vi "诊断标定3.vi"(8 "CAN端口":u16(ring), 9 "设备索引号":u16(ring), 10 "CAN卡类型":u32(ring)=21) -> ()   [LabVIEW 2013] (continued)
                        n4317 = Build Array(string[] ["电池生产日期", "电池厂商", "电池类型", "电池包组号", "电池包产权标识", "电池包应用车型", "电池串联", "电池并联", "累计充电总安时", "累计放电总安时", "电池包额定容量", "电池包额定能量", "电池包额定总电压", "电池充满次数", "电池放空次数", "电池充电次数", "实际容量"], w6126) -> (w6147:string[][])
                        n4318 = Transpose 2D Array(2D array=w6147) -> (transposed array=w6125:string[][])
                      }
                    }
                    n4319 = Insert Into Array(array=w5966, index (col)=2 ("禁用的索引 (列)"), new element #1=w5963, new element #2=w5962, new element #3=w5961, new element #4=w5960, new element #5=w5959) -> (w5964:string[][])  [unwired: 1 in]
                  }
                  frame "从板" {
                    n4320 = local read "从板号"() -> (w6163:u8)
                    n4321 = Number To Decimal String(number=w6163) -> (decimal integer string=w6160:string)  [unwired: 1 out]
                    n4322 = Concatenate Strings("S", w6160) -> (w6161:string)
                    n4323 = Build Array("从板号" ("元素"), w6160) -> (w6158:string[])
                    n4324 = stacked-sequence {
                      seq-local: [string[] ["风机开启温度", "风机关闭温度", "加热开启温度", "加热关闭温度", "风机开启温差", "风机关闭温差", "加热关闭温差"] _ _ _ _ _] -> [_ _ _ w6232 _ _]
                      seq-local: [w6175 _ _ _ _ _] -> [_ _ _ w6228 _ _]
                      seq-local: [_ string[] ["电压过高一级", "电压过低一级", "温度过高一级", "温度过低一级", "电压不均衡一级", "温度不均衡一级", "SOC过低一级"] _ _ _ _] -> [_ _ _ w6231 _ _]
                      seq-local: [_ w6193 _ _ _ _] -> [_ _ _ w6227 _ _]
                      seq-local: [_ _ string[] ["电压过高二级", "电压过低二级", "温度过高二级", "温度过低二级", "电压不均衡二级", "温度不均衡二级", "SOC过低二级"] _ _ _] -> [_ _ _ w6230 _ _]
                      seq-local: [_ _ w6208 _ _ _] -> [_ _ _ w6226 _ _]
                      tunnel: w6158 -> [w6188 _ _ _ _ _]
                      tunnel: [w6177 _ _ _ _ _] -> w6156
                      tunnel: [_ _ _ w6233 _ _] -> w6154
                      tunnel: [_ _ _ _ w6271 _] -> w6153
                      tunnel: [_ _ _ _ _ w6307] -> _
                      frame #0 {
                        w6168 = string[] ["", "", "", "", "", "", "", "", "", "", "  "]
                        n4325 = control-ref of="项目信息 2"() -> (w6187:refnum<vi>)
                        n4326 = property class="Tbl (严格)"(reference=w6187) -> ("Value"=w6165:string[][])  [unwired: 1 in, 2 out]
                        n4327 = control-ref of="加热控制参数"() -> (w6179:refnum<vi>)
                        n4328 = property class="Clust (严格)"(reference=w6179) -> ("Value"=w6186:T11)  [unwired: 1 in, 2 out]
                        n4329 = Unbundle(w6186) -> ("风机开启温度"=w6185:dbl, "风机关闭温度"=w6184:dbl, "加热开启温度"=w6183:dbl, "加热关闭温度"=w6182:dbl, "风机开启温差"=w6181:dbl, "风机关闭温差"=w6180:dbl, "加热关闭温差"=w6174:dbl)
                        n4330 = Build Array(w6185, w6184, w6183, w6182, w6181, w6180, w6174) -> (w6178:dbl[])
                        n4331 = for {
                          tunnel: w6178 -> [w6191] mode=indexing
                          tunnel: [w6190] -> w6175 mode=indexing
                          n4332 = Format Into String(format string="%#f" ("格式字符串"), w6191) -> (resulting string=w6190:string)  [unwired: 2 in, 1 out]
                        }
                        n4333 = Index Array(array=w6165, index (col)=0 ("禁用的索引 (列)")) -> (element=w6172:string[])  [unwired: 1 in]
                        n4334 = Index Array(array=w6165, index (col)=1 ("禁用的索引 (列)")) -> (element=w6171:string[])  [unwired: 1 in]
                        n4335 = Insert Into Array(array=w6172, new element=w6168) -> (w6170:string[])  [unwired: 1 in]
                        n4336 = Insert Into Array(array=w6171, new element=w6168) -> (w6169:string[])  [unwired: 1 in]
                        n4337 = Build Array(w6170, w6169) -> (w6166:string[][])
                        n4338 = Transpose 2D Array(2D array=w6166) -> (transposed array=w6164:string[][])
                        n4339 = Insert Into Array(array=w6164, index (row)=0 ("索引 (行)"), new element=w6188) -> (w6177:string[][])  [unwired: 1 in]
                      }
                      frame #1 {
                        n4340 = control-ref of="一级故障(从板)"() -> (w6204:refnum<vi>)
                        n4341 = property class="Clust (严格)"(reference=w6204) -> ("Value"=w6203:T15)  [unwired: 1 in, 2 out]
                        n4342 = Unbundle(w6203) -> ("电压过高"=w6202:dbl, "电压过低"=w6201:dbl, "温度过高"=w6200:dbl, "温度过低"=w6199:dbl, "电压不均衡(V)"=w6198:dbl, "温度不均衡"=w6197:dbl, "SOC过低"=w6196:dbl)
                        n4343 = Build Array(w6202, w6201, w6200, w6199, w6198, w6197, w6196) -> (w6195:dbl[])
                        n4344 = for {
                          tunnel: w6195 -> [w6206] mode=indexing
                          tunnel: [w6205] -> w6193 mode=indexing
                          n4345 = Format Into String(format string="%#f" ("格式字符串"), w6206) -> (resulting string=w6205:string)  [unwired: 2 in, 1 out]
                        }
                      }
                      frame #2 {
                        n4346 = control-ref of="二级故障(从板)"() -> (w6210:refnum<vi>)
                        n4347 = property class="Clust (严格)"(reference=w6210) -> ("Value"=w6219:T15)  [unwired: 1 in, 2 out]
                        n4348 = Unbundle(w6219) -> ("电压过高"=w6218:dbl, "电压过低"=w6217:dbl, "温度过高"=w6216:dbl, "温度过低"=w6215:dbl, "电压不均衡(V)"=w6214:dbl, "温度不均衡"=w6213:dbl, "SOC过低"=w6212:dbl)
                        n4349 = Build Array(w6218, w6217, w6216, w6215, w6214, w6213, w6212) -> (w6211:dbl[])
                        n4350 = for {
                          tunnel: w6211 -> [w6221] mode=indexing
                          tunnel: [w6220] -> w6208 mode=indexing
                          n4351 = Format Into String(format string="%#f" ("格式字符串"), w6221) -> (resulting string=w6220:string)  [unwired: 2 in, 1 out]
                        }
                      }
                      frame #3 {
                        n4352 = control-ref of="三级故障(从板)"() -> (w6234:refnum<vi>)
                        n4353 = property class="Clust (严格)"(reference=w6234) -> ("Value"=w6244:T15)  [unwired: 1 in, 2 out]
                        n4354 = Unbundle(w6244) -> ("电压过高"=w6243:dbl, "电压过低"=w6242:dbl, "温度过高"=w6241:dbl, "温度过低"=w6240:dbl, "电压不均衡(V)"=w6239:dbl, "温度不均衡"=w6238:dbl, "SOC过低"=w6237:dbl)
                        n4355 = Build Array(w6243, w6242, w6241, w6240, w6239, w6238, w6237) -> (w6236:dbl[])
                        n4356 = for {
                          tunnel: w6236 -> [w6246] mode=indexing
                          tunnel: [w6245] -> w6225 mode=indexing
                          n4357 = Format Into String(format string="%#f" ("格式字符串"), w6246) -> (resulting string=w6245:string)  [unwired: 2 in, 1 out]
                        }
                        n4358 = Insert Into Array(array=w6232, new element #1=w6231, new element #2=w6230, new element #3=string[] ["电压过高三级", "电压过低三级", "温度过高三级", "温度过低三级", "电压不均衡三级", "温度不均衡三级", "SOC过低三级"]) -> (w6223:string[])  [unwired: 1 in]
                        n4359 = Insert Into Array(array=w6228, new element #1=w6227, new element #2=w6226, new element #3=w6225) -> (w6224:string[])  [unwired: 1 in]
                        n4360 = Build Array(w6223, w6224) -> (w6235:string[][])
                        n4361 = Transpose 2D Array(2D array=w6235) -> (transposed array=w6233:string[][])
                      }
                      frame #4 {
                        n4362 = control-ref of="快换(从板)"() -> (w6270:refnum<vi>)
                        n4363 = property class="Clust (严格)"(reference=w6270) -> ("Value"=w6283:T16)  [unwired: 1 in, 2 out]
                        n4364 = Unbundle(w6283) -> ("串联数"=w6282:dbl, "并联数"=w6281:dbl, "电池厂家"=w6280:dbl, "电池类型"=w6279:dbl, "额定能量"=w6278:dbl, "额定容量"=w6277:dbl, "实际容量"=w6276:dbl, "额定总压"=w6269:dbl, "产权标识"=w6268:dbl, "应用车型"=w6267:dbl, "电池包组号"=w6266:dbl, "SOC"=w6264:dbl, "充电总安时"=w6263:dbl, "放电总安时"=w6262:dbl, "放空次数"=w6261:dbl, "充满次数"=w6260:dbl, "充电次数"=w6259:dbl, "车牌号"=w6249:string, "生产日期"=w6248:string, "最大允许单体电压"=w6258:dbl, "最大允许总电压"=w6257:dbl, "最大允许温度"=w6256:dbl, "最小允许温度"=w6255:dbl, "最大允许充电电流"=w6254:dbl, "最小允许充电电流"=w6253:dbl, "最小允许单体电压"=w6252:dbl, "电流步长"=w6251:dbl, "电池包序号"=w6250:dbl)
                        n4365 = Build Array(w6282, w6281, w6280, w6279, w6278, w6277, w6276, w6269, w6268, w6267, w6266, w6264, w6263, w6262, w6261, w6260, w6259, w6258, w6257, w6256, w6255, w6254, w6253, w6252, w6251, w6250) -> (w6275:dbl[])
                        n4366 = for {
                          tunnel: w6275 -> [w6285] mode=indexing
                          tunnel: [w6284] -> w6273 mode=indexing
                          n4367 = Format Into String(format string="%#f" ("格式字符串"), w6285) -> (resulting string=w6284:string)  [unwired: 2 in, 1 out]
                        }
                        n4368 = Insert Into Array(array=w6273, new element #1=w6249, new element #2=w6248) -> (w6265:string[])  [unwired: 1 in]
                        n4369 = call <vilib>:"Unset Busy.vi"() -> ()  [unwired: 2 in, 10 out]
                        n4370 = Build Array(string[] ["电池串联数", "电池并联数", "电池厂家", "额定能量", "额定容量", "实际容量", "额定总压", "产权标识", "应用车型", "电池包组号", "SOC", "充电总安时", "放电总安时", "放空次数", "充满次数", "充电次数", "最大允许单体电压", "最大允许总电压", "最大允许温度", "最小允许温度", "最大允许充电电流", "最小允许充电电流", "最小允许单体电压", "电流步长", "电池包序号"], w6265) -> (w6274:string[][])
                        n4371 = Transpose 2D Array(2D array=w6274) -> (transposed array=w6271:string[][])
                      }
                      frame #5 {
                        n4372 = local read "均衡参数"() -> (w6306:T17)
                        n4373 = Unbundle(w6306) -> ("充电结束电压(90%)"=w6298:sgl, "充电结束电压(91%)"=w6297:sgl, "充电结束电压(92%)"=w6296:sgl, "充电结束电压(93%)"=w6295:sgl, "充电结束电压(94%)"=w6294:sgl, "均衡计算-电压高阀值1级"=w6305:sgl, "均衡计算-电压高阀值2级"=w6304:sgl, "均衡计算-电压低阀值1级"=w6303:sgl, "均衡计算-电压低阀值2级"=w6302:sgl, "均衡计算-最低电压阀值"=w6301:sgl, "均衡停止-最低电压阀值"=w6300:sgl, "均衡计算-电压极差阀值"=w6299:sgl, "充电结束电压(95%)"=w6293:sgl, "充电结束电压(96%)"=w6292:sgl, "充电结束电压(97%)"=w6291:sgl, "充电结束电压(98%)"=w6290:sgl, "充电结束电压(99%)"=w6289:sgl, "充电结束电压(100%)"=w6288:sgl)
                        n4374 = Build Array(w6305, w6304, w6303, w6302, w6301, w6300, w6299, w6298, w6297, w6296, w6295, w6294, w6293, w6292, w6291, w6290, w6289, w6288) -> (w6310:sgl[])
                        n4375 = for {
                          tunnel: w6310 -> [w6312] mode=indexing
                          tunnel: [w6311] -> w6287 mode=indexing
                          n4376 = Format Into String(format string="%#f" ("格式字符串"), w6312) -> (resulting string=w6311:string)  [unwired: 2 in, 1 out]
                        }
                        n4377 = call <vilib>:"Unset Busy.vi"() -> ()  [unwired: 2 in, 10 out]
                        n4378 = Build Array(string[] ["均衡计算-电压高阀值1级", "均衡计算-电压高阀值2级", "均衡计算-电压低阀值1级", "均衡计算-电压低阀值2级", "均衡计算-最低电压阀值", "均衡停止-最低电压阀值", "均衡计算-电压极差阀值", "充电结束电压(90%)", "充电结束电压(91%)", "充电结束电压(92%)", "充电结束电压(93%)", "充电结束电压(94%)", "充电结束电压(95%)", "充电结束电压(96%)", "充电结束电压(97%)", "充电结束电压(98%)", "充电结束电压(99%)", "充电结束电压(100%)"], w6287) -> (w6309:string[][])
                        n4379 = Transpose 2D Array(2D array=w6309) -> (transposed array=w6307:string[][])
                      }
                    }
                    n4380 = Insert Into Array(array=w6156, index (col)=2 ("禁用的索引 (列)"), new element #1=w6154, new element #2=w6153) -> (w6155:string[][])  [unwired: 1 in]
                  }
                }
                n4381 = call "当前时间解析-8.6.vi"() -> ("名称格式时间"=w5947:string)  [unwired: 1 in, 18 out]
                n4382 = Concatenate Strings(w5947, w5946, ".txt" ("字符串")) -> (w5944:string)
                n4383 = call "自适应屏幕分辨率.vi"() -> ()  [unwired: 16 in]
                n4384 = call "文件对话框2"("prompt"="选择保存的路径", "default name"=w5944, "pattern (all files)"="*.txt") -> ("selected path"=w5942:path, "cancelled"=w5941:bool, "error out"=w5940:errorcluster)  [unwired: 9 in, 1 out]
                n4385 = call <vilib>:"Clear Errors.vi"("error in (no error)"=w5940) -> ()  [unwired: 6 in, 1 out]
                n4386 = case shown="假" w5941 {
                  tunnel: w5948 -> [w5953 _]
                  tunnel: w5942 -> [w5949 _]
                  frame False {
                    n4387 = call-poly <vilib>:"Write To Spreadsheet File.vi"("append to file? (new file:F)"=FALSE, "2D data"=w5953, "file path (dialog if empty)"=w5949) -> ("new file path (Not A Path if cancelled)"=w5951:path)  [unwired: 3 in, 2 out]
                    n4388 = Path To String(path=w5951) -> (string=w5950:string)
                    n4389 = stacked-sequence {
                      tunnel: w5950 -> [w5956]
                      frame #0 {
                        n4390 = Concatenate Strings("保存完成,路径为:" ("字符串"), w5956) -> (w5957:string)
                        n4391 = One Button Dialog(message=w5957, button name ("OK")="是" ("按钮名称（“确定”）")) -> ()  [unwired: 1 out]
                      }
                    }
                  }
                  frame True {
                  }
                }
              }
              frame Disabled {
                n4392 = stacked-sequence {
                  seq-local: [w6327] -> [_]
                  frame #0 {
                    n4393 = local read "项目信息"() -> (w6329:string[][])
                    n4394 = local read "项目信息2"() -> (w6326:T9)
                    n4395 = Array Subset(array=w6329, index (row)=0 ("索引"), index (col)=0 ("索引"), length (col)=2 ("索引")) -> (w6332:string[][])  [unwired: 1 in]
                    n4396 = local read "一级故障"() -> ()  [unwired: 1 out]
                    n4397 = local read "从板个数"() -> (w6327:dbl)
                    n4398 = Unbundle(w6326) -> ("电池额定容量(A)"=w6325:dbl, "电池实际容量(A)"=w6324:dbl, "车架(牌)号"=w6318:string, "配置文件版本"=w6317:string, "SOH(%)"=w6322:dbl, "SOC(%)"=w6323:dbl, "产品编号"=w6319:string)  [unwired: 2 out]
                    n4399 = Index Array(array=w6332, index (col) #1=1 ("禁用的索引 (列)"), index (col) #2=0 ("索引 (列)")) -> (element #1=w6316:string[], element #2=w6315:string[])  [unwired: 2 in]
                    n4400 = Build Array(w6325, w6324, w6323, w6322) -> (w6321:dbl[])
                    n4401 = Number To Decimal String(number=w6327) -> ()  [unwired: 1 in, 1 out]
                    n4402 = for {
                      tunnel: w6321 -> [w6337] mode=indexing
                      tunnel: [w6336] -> w6320 mode=indexing
                      n4403 = Format Into String(format string="%#f" ("格式字符串"), w6337) -> (resulting string=w6336:string)  [unwired: 2 in, 1 out]
                    }
                    n4404 = Insert Into Array(array=w6320, new element #1=w6319, new element #2=w6318, new element #3=w6317, new element #4=w6316) -> ()  [unwired: 1 in, 1 out]
                    n4405 = Insert Into Array(array=string[] ["电池额定容量", "电池实际容量", "SOC", "SOH", "产品编号", "车架(牌)号", "配置文件版本"], new element=w6315) -> ()  [unwired: 1 in, 1 out]
                  }
                }
              }
            }
          }
          frame "读配置文件" {
            n4406 = local read "主从选择"() -> (w6350:enum32{"主板", "从板"})
            n4407 = case shown="\"主板\", 默认" w6350 {
              tunnel: ["M" ("pattern (all files)") "S" ("pattern (all files)")] -> _
              tunnel: ["主板" ("pattern (all files)") "从板" ("pattern (all files)")] -> w6349
              frame "主板", Default {
              }
              frame "从板" {
              }
            }
            n4408 = case shown="真" "布尔" {
              tunnel: [w6752 w6757] -> w6342
              tunnel: [FALSE ("cancelled") w6756] -> _
              tunnel: w6349 -> [_ w6755]
              frame False {
                n4409 = local read "路径"() -> (w6752:path)
              }
              frame True {
                n4410 = global read "配置文件全局.vi" "诊断标定读取地址"() -> (w6753:path)
                n4411 = call "文件对话框"("start path"=w6753, "prompt"="选择要读取的配置文件", "button label"=w6755) -> ("selected path"=w6757:path, "cancelled"=w6756:bool, "error out"=w6754:errorcluster)  [unwired: 4 in, 6 out]
                n4412 = call <vilib>:"Clear Errors.vi"("error in (no error)"=w6754) -> ()  [unwired: 7 out]
              }
            }
            n4413 = Strip Path(path=w6342) -> (stripped path=w6338:path, name=w6346:string)
            n4414 = Match Pattern(string=w6346, regular expression=".ini" ("正则表达式")) -> (offset past match=w6344:i32)  [unwired: 1 in, 3 out]
            n4415 = control-ref of="结果"() -> (w6348:refnum<vi>)
            n4416 = global write "配置文件全局.vi" "诊断标定读取地址"(w6338) -> ()
            n4417 = Not Equal?(x=w6344, y=-1) -> (x != y?=w6339:bool)
            n4418 = case shown="真" w6339 {
              tunnel: w6342 -> [_ w6359]
              tunnel: [_ w6368] -> w6340
              frame False {
              }
              frame True {
                w6371 = "MD5码" ("key")
                w6372 = "总信息" ("section")
                n4419 = Strip Path(path=w6359) -> (stripped path=w6357:path, name=w6356:string)
                n4420 = Match Pattern(string=w6356, regular expression=".ini" ("正则表达式")) -> (before substring=w6353:string, match substring=w6354:string)  [unwired: 1 in, 2 out]
                n4421 = Concatenate Strings(w6353, "-rc" ("字符串"), w6354) -> (w6352:string)
                n4422 = Build Path(base path=w6357, name or relative path=w6352) -> (appended path=w6358:path)
                n4423 = Copy(10:w6358, 11:w6359) -> (3:w6363:path)  [unwired: 3 in, 2 out]
                n4424 = call <vilib>:"Open Config Data.vi"("create file if necessary (T)"=FALSE, "configuration file path"=w6363) -> ("refnum"=w6374:T25)  [unwired: 7 in, 2 out]
                n4425 = call-poly <vilib>:"Read Key.vi"("section"=w6372, "key"=w6371, "refnum"=w6374) -> ("value"=w6369:string, "refnum out"=w6373:T25)  [unwired: 5 in, 2 out]
                n4426 = call-poly <vilib>:"Write Key.vi"("section"=w6372, "value"=w6371, "key"=w6371, "refnum"=w6373) -> ("error out"=w6367:errorcluster, "found?"=w6366:bool, "refnum out"=w6365:T25)  [unwired: 5 in]
                n4427 = call <vilib>:"Close Config Data.vi"("error in (no error)"=w6367, "write file if changed (T)"=w6366, "refnum"=w6365) -> ("error out"=w6364:errorcluster, "file path"=w6361:path)  [unwired: 7 in]
                n4428 = call <vilib>:"MD5Checksum File.vi"("error in (no error)"=w6364, "Path"=w6361) -> ("error out"=w6362:errorcluster, "MD5 message-digest"=w6370:string)  [unwired: 8 in]
                n4429 = Equal?(x=w6370, y=w6369) -> (x = y?=w6368:bool)
                n4430 = Delete(path (use dialog)=w6361, error in=w6362) -> (error out=w6360:errorcluster)  [unwired: 3 in, 2 out]
                n4431 = call <vilib>:"Clear Errors.vi"("error in (no error)"=w6360) -> ()  [unwired: 6 in, 1 out]
              }
            }
            n4432 = And(x=w6339, y=w6340) -> (x .and. y?=w6341:bool)
            n4433 = case shown="真" w6341 {
              tunnel: w6342 -> [_ w6392]
              tunnel: w6348 -> [w6378 w6391]
              tunnel: w6340 -> [w6377 _]
              tunnel: w6339 -> [w6376 _]
              frame False {
                n4434 = stacked-sequence {
                  tunnel: w6376 -> [w6380 _]
                  tunnel: w6378 -> [w6379 w6386]
                  tunnel: w6377 -> [_ w6385]
                  frame #0 {
                    n4435 = case shown="假" w6380 {
                      tunnel: w6379 -> [w6382 _]
                      frame False {
                        n4436 = Build Array("文件格式错误") -> (w6383:string[])
                        n4437 = call "表格编辑.vi"("新元素/子数组"=w6383, "活动单元格:单元格背景色"=u32 16711680, "MCListbox引用句柄"=w6382) -> ()  [unwired: 9 out]
                      }
                      frame True {
                      }
                    }
                  }
                  frame #1 {
                    n4438 = case shown="假" w6385 {
                      tunnel: w6386 -> [w6388 _]
                      frame False {
                        n4439 = Build Array("文件MD5码验证错误") -> (w6389:string[])
                        n4440 = call "表格编辑.vi"("新元素/子数组"=w6389, "活动单元格:单元格背景色"=u32 16711680, "MCListbox引用句柄"=w6388) -> ()  [unwired: 9 out]
                      }
                      frame True {
                      }
                    }
                  }
                }
                n4441 = call <vilib>:"Unset Busy.vi"() -> ()  [unwired: 11 in, 1 out]
              }
              frame True {
                n4442 = stacked-sequence {
                  seq-local: [w6397 _ _ _] -> [_ w6625 w6719 _]
                  seq-local: [w6395 _ _ _] -> [_ w6603 _ _]
                  tunnel: w6392 -> [w6393 _ _ _]
                  tunnel: w6391 -> [w6410 _ _ w6746]
                  frame #0 {
                    w6394 = string[][] []
                    w6407 = "总信息" ("section")
                    n4443 = local write "路径"(w6393) -> ()
                    n4444 = call <vilib>:"Open Config Data.vi"("create file if necessary (T)"=FALSE, "configuration file path"=w6393) -> ("error out"=w6398:errorcluster, "refnum"=w6397:T25)  [unwired: 7 in, 1 out]
                    n4445 = call <vilib>:"Get Key Names.vi"("section"=w6407, "error in (no error)"=w6398, "refnum"=w6397) -> ("key names"=w6406:string[], "refnum out"=w6408:T25)  [unwired: 5 in, 2 out]
                    n4446 = for {
                      tunnel: w6408 -> [w6414]
                      tunnel: w6407 -> [w6413]
                      tunnel: w6406 -> [w6412] mode=indexing
                      tunnel: [w6411] -> w6403 mode=indexing
                      n4447 = call-poly <vilib>:"Read Key.vi"("section"=w6413, "key"=w6412, "refnum"=w6414) -> ("value"=w6411:string)  [unwired: 5 in, 3 out]
                    }
                    n4448 = Index Array(array=w6403) -> (element #1=w6396:string, element #2=w6401:string)  [unwired: 2 in]
                    n4449 = Decimal String To Number(string=w6396) -> (number=w6395:i32)  [unwired: 2 in, 1 out]
                    n4450 = Concatenate Strings("正在读取" ("字符串"), w6401, "的配置文件" ("字符串")) -> (w6399:string)
                    n4451 = Build Array(w6399) -> (w6404:string[])
                    n4452 = call "表格编辑.vi"("新元素/子数组"=w6404, "活动单元格:单元格背景色"=u32 6618880, "MCListbox引用句柄"=w6410) -> ()  [unwired: 9 out]
                    n4453 = local write "项目信息"(w6394) -> ()
                    n4454 = local write "项目信息 2"(w6394) -> ()
                  }
                  frame #1 {
                    w6585 = 20 ("长度")
                    w6626 = "主板" ("section")
                    n4455 = call <vilib>:"Get Key Names.vi"("section"=w6626, "refnum"=w6625) -> ("key names"=w6427:string[], "refnum out"=w6627:T25)  [unwired: 6 in, 2 out]
                    n4456 = for {
                      tunnel: w6627 -> [w6639]
                      tunnel: w6626 -> [w6638]
                      tunnel: w6427 -> [w6637] mode=indexing
                      tunnel: [w6636] -> w6426 mode=indexing
                      n4457 = call-poly <vilib>:"Read Key.vi"("section"=w6638, "key"=w6637, "refnum"=w6639) -> ("value"=w6636:string)  [unwired: 5 in, 3 out]
                    }
                    n4458 = Search 1D Array(1D array=w6427, element="总电压过高一级" ("元素"), start index (0)=0 ("开始索引(0)")) -> (index of element=w6507:i32)
                    n4459 = Search 1D Array(1D array=w6427, element="风机开启温度" ("元素"), start index (0)=w6507) -> (index of element=w6498:i32)
                    n4460 = Search 1D Array(1D array=w6427, element="电池串联" ("元素"), start index (0)=w6498) -> (index of element=w6496:i32)
                    n4461 = Decrement(x=w6507) -> (x-1=w6624:i32)
                    n4462 = Array Subset(array=w6427, index=1 ("索引"), length=w6624) -> (w6472:string[])
                    n4463 = Array Subset(array=w6426, index=1 ("索引"), length=w6624) -> (w6469:string[])
                    n4464 = Delete From Array(array=w6469, length=7 ("长度"), index=0 ("索引")) -> (deleted portion=w6466:string[], array with subset deleted=w6416:string[])
                    n4465 = Delete From Array(array=w6472, length=7 ("长度"), index=0 ("索引")) -> (array with subset deleted=w6425:string[])  [unwired: 1 out]
                    n4466 = Search 1D Array(1D array=w6427, element="分流器型号" ("元素")) -> (index of element=w6430:i32)  [unwired: 1 in]
                    n4467 = Index Array(array=w6426, index=0 ("索引")) -> (element=w6600:string)
                    n4468 = Decimal String To Number(string=w6600) -> (number=w6417:i32)  [unwired: 2 in, 1 out]
                    n4469 = Search 1D Array(1D array=w6425, element="主板电池节数" ("元素")) -> (index of element=w6591:i32)  [unwired: 1 in]
                    n4470 = Search 1D Array(1D array=w6425, element="主板温度起始值" ("元素")) -> (index of element=w6588:i32)  [unwired: 1 in]
                    n4471 = Search 1D Array(1D array=w6425, element="第一个保险通道" ("元素")) -> (index of element=w6587:i32)  [unwired: 1 in]
                    n4472 = Search 1D Array(1D array=w6425, element="主板温度个数" ("元素")) -> (index of element=w6589:i32)  [unwired: 1 in]
                    n4473 = Search 1D Array(1D array=w6425, element="主板电压起始值" ("元素")) -> (index of element=w6590:i32)  [unwired: 1 in]
                    n4474 = Search 1D Array(1D array=w6425, element="第1通道电压个数" ("元素")) -> (index of element=w6586:i32)  [unwired: 1 in]
                    n4475 = Index Array(array=w6426, index=w6430) -> (element=w6429:string)
                    n4476 = for {
                      N: 4 -> [_]
                      tunnel: w6466 -> [w6635] mode=indexing
                      tunnel: [w6634] -> w6615 mode=indexing
                      n4477 = Fract/Exp String To Number(string=w6635) -> (number=w6634:dbl)  [unwired: 3 in, 1 out]
                    }
                    n4478 = Increment(x=w6417) -> (x+1=w6599:i32)
                    n4479 = Increment(x=w6417) -> (x+1=w6584:i32)
                    n4480 = Increment(x=w6417) -> (x+1=w6597:i32)
                    n4481 = Increment(x=w6417) -> (x+1=w6598:i32)
                    n4482 = global write "读配置文件全局.vi" "从板个数"(w6417) -> ()
                    n4483 = local write "从板个数"(w6417) -> ()
                    n4484 = Decimal String To Number(string=w6429) -> (number=w6428:i32)  [unwired: 2 in, 1 out]
                    n4485 = Index Array(array=w6466, index #1=4 ("索引"), index #2=5 ("索引"), index #3=6 ("索引")) -> (element #1=w6606:string, element #2=w6605:string, element #3=w6604:string)
                    n4486 = Index Array(array=w6615) -> (element #1=w6613:dbl, element #2=w6612:dbl, element #3=w6611:dbl, element #4=w6610:dbl)  [unwired: 4 in]
                    n4487 = global write "EV05全局变量1.vi" "分流器型号"(w6428) -> ()
                    n4488 = Array Subset(array=w6416, index=w6591, length=w6599) -> (w6583:string[])
                    n4489 = Array Subset(array=w6416, index=w6590, length=w6598) -> (w6581:string[])
                    n4490 = Array Subset(array=w6416, index=w6589, length=w6597) -> (w6580:string[])
                    n4491 = Array Subset(array=w6416, index=w6588, length=w6584) -> (w6579:string[])
                    n4492 = Array Subset(array=w6416, index=w6587, length=20 ("长度")) -> (w6578:string[])
                    n4493 = Array Subset(array=w6416, index=w6586, length=w6585) -> (w6582:string[])
                    n4494 = Multiply(x=w6417, y=2) -> (x*y=w6418:i32)
                    n4495 = control-ref of="项目信息2"() -> (w6618:refnum<vi>)
                    n4496 = Array Subset(array=w6416, index=0 ("索引"), length=w6418) -> (w6415:string[])
                    n4497 = Insert Into Array(array=w6583, new element #1=w6582, new element #2=w6581, new element #3=w6580, new element #4=w6579, new element #5=w6578) -> ()  [unwired: 1 in, 1 out]
                    n4498 = property class="Clust (严格)"(reference=w6618) -> (reference out=w6616:refnum<vi>, "Value"=w6617:T9)  [unwired: 1 in, 1 out]
                    n4499 = Multiply(x=w6417, y=2) -> (x*y=w6422:i32)
                    n4500 = Array Subset(array=w6425, index=w6591, length=w6584) -> (w6456:string[])
                    n4501 = Array Subset(array=w6425, index=w6590, length=w6584) -> (w6454:string[])
                    n4502 = Array Subset(array=w6425, index=w6589, length=w6584) -> (w6453:string[])
                    n4503 = Array Subset(array=w6425, index=w6588) -> (w6452:string[])  [unwired: 1 in]
                    n4504 = Array Subset(array=w6425, index=w6587, length=w6585) -> (w6451:string[])
                    n4505 = Array Subset(array=w6425, index=w6586, length=w6585) -> (w6455:string[])
                    n4506 = Array Subset(array=w6425, index=0 ("索引"), length=w6422) -> (w6421:string[])
                    n4507 = global write "读配置文件全局.vi" "表格输入"(w6415) -> ()
                    n4508 = Build Array(w6421, w6415) -> (w6577:string[][])
                    n4509 = Bundle(cluster=w6617, "电池额定容量(A)"=w6613, "使用者"=w6603, "电池实际容量(A)"=w6612, "车架(牌)号"=w6605, "配置文件版本"=w6604, "SOH(%)"=w6610, "SOC(%)"=w6611, "产品编号"=w6606) -> (w6443:T9)  [unwired: 1 in]
                    n4510 = Transpose 2D Array(2D array=w6577) -> (transposed array=w6444:string[][])
                    n4511 = Multiply(x=w6417, y=4) -> (x*y=w6448:i32)
                    n4512 = Insert Into Array(array=w6456, new element #1=w6455, new element #2=w6454, new element #3=w6453, new element #4=w6452, new element #5=w6451) -> (w6450:string[])  [unwired: 1 in]
                    n4513 = Add(x=w6448, y=44) -> (x+y=w6446:i32)
                    n4514 = local write "项目信息"(w6444) -> ()
                    n4515 = property class="Clust (严格)"(reference=w6616, "Value"=w6443) -> ()  [unwired: 1 in, 2 out]
                    n4516 = global write "读配置文件全局.vi" "项目信息"(w6443) -> ()
                    n4517 = Array Subset(array=w6426, index=w6496, length=15 ("长度")) -> (w6434:string[])
                    n4518 = Array Subset(array=w6450, index=0 ("索引"), length=w6446) -> ()  [unwired: 1 out]
                    n4519 = Array Subset(array=w6426, index=w6498, length=15 ("长度")) -> (w6503:string[])
                    n4520 = Delete From Array(array=w6434, length=4 ("长度"), index=6 ("索引")) -> (deleted portion=w6490:string[], array with subset deleted=w6489:string[])
                    n4521 = for {
                      tunnel: w6503 -> [w6631] mode=indexing
                      tunnel: [w6630] -> w6502 mode=indexing
                      n4522 = Fract/Exp String To Number(string=w6631) -> (number=w6630:dbl)  [unwired: 3 in, 1 out]
                    }
                    n4523 = for {
                      tunnel: w6489 -> [w6629] mode=indexing
                      tunnel: [w6628] -> w6488 mode=indexing
                      n4524 = Fract/Exp String To Number(string=w6629) -> (number=w6628:dbl)  [unwired: 3 in, 1 out]
                    }
                    n4525 = Array Subset(array=w6426, index=w6507, length=51 ("长度")) -> (w6576:string[])
                    n4526 = for {
                      tunnel: w6576 -> [w6633] mode=indexing
                      tunnel: [w6632] -> w6575 mode=indexing
                      n4527 = Fract/Exp String To Number(string=w6633) -> (number=w6632:dbl)  [unwired: 3 in, 1 out]
                    }
                    n4528 = Index Array(array=w6488) -> (element #1=w6483:dbl, element #2=w6482:dbl, element #3=w6481:dbl, element #4=w6480:dbl, element #5=w6479:dbl, element #6=w6478:dbl, element #7=w6477:dbl, element #8=w6476:dbl, element #9=w6475:dbl, element #10=w6474:dbl, element #11=w6473:dbl)  [unwired: 11 in]
                    n4529 = Delete From Array(array=w6502, length=7 ("长度"), index=0 ("索引")) -> (deleted portion=w6439:dbl[], array with subset deleted=w6500:dbl[])
                    n4530 = Delete From Array(array=w6575, length=17 ("长度"), index=0 ("索引")) -> (deleted portion=w6436:dbl[], array with subset deleted=w6572:dbl[])
                    n4531 = Array To Cluster(array=w6439) -> (cluster=w6501:T26)
                    n4532 = global write "读配置文件全局.vi" "加热控制参数"(w6439) -> ()
                    n4533 = Index Array(array=w6500) -> (element #1=w6464:dbl, element #2=w6463:dbl, element #3=w6462:dbl, element #4=w6461:dbl, element #5=w6460:dbl, element #6=w6459:dbl, element #7=w6458:dbl, element #8=w6457:dbl)  [unwired: 8 in]
                    n4534 = Delete From Array(array=w6572, length=17 ("长度"), index=0 ("索引")) -> (deleted portion=w6435:dbl[], array with subset deleted=w6432:dbl[])
                    n4535 = Index Array(array=w6490) -> (element #1=w6487:string, element #2=w6486:string, element #3=w6484:string, element #4=w6485:string)  [unwired: 4 in]
                    n4536 = local write "加热控制参数"(w6501) -> ()
                    n4537 = global write "读配置文件全局.vi" "一级故障"(w6436) -> ()
                    n4538 = local read "一级故障 5"() -> (w6465:T12)
                    n4539 = control-ref of="电池信息"() -> (w6494:refnum<vi>)
                    n4540 = global write "读配置文件全局.vi" "二级故障"(w6435) -> ()
                    n4541 = global write "读配置文件全局.vi" "三级故障"(w6432) -> ()
                    n4542 = Bundle(cluster=w6465, "最大允许单体电压"=w6464, "最大允许总电压"=w6460, "最小允许单体电压"=w6463, "最大允许充电电流"=w6462, "最小允许充电电流"=w6461, "最大允许充电温度"=w6459, "最小允许充电温度"=w6458, "电流步长"=w6457) -> (w6438:T12)
                    n4543 = property class="Clust (严格)"(reference=w6494) -> (reference out=w6495:refnum<vi>, "Value"=w6493:T13)  [unwired: 1 in, 1 out]
                    n4544 = Bundle(cluster=w6493, "电池串联"=w6483, "电池并联"=w6482, "累计放电总安时"=w6476, "电池包额定容量"=w6481, "电池包额定能量(kWh)"=w6480, "电池包额定总电压"=w6479, "累计充电总安时"=w6477, "电池充满次数"=w6474, "电池放空次数"=w6475, "电池充电次数"=w6473, "电池生产日期"=w6484, "电池厂家"=w6487, "电池类型"=w6486, "电池包组号"=w6485, "实际容量"=w6478) -> (w6433:T13)  [unwired: 2 in]
                    n4545 = Cluster To Array(cluster=w6438) -> (array=w6437:dbl[])
                    n4546 = local write "一级故障 5"(w6438) -> ()
                    n4547 = global write "读配置文件全局.vi" "充电控制参数"(w6437) -> ()
                    n4548 = Index Array(array=w6436) -> (element #1=w6565:dbl, element #2=w6564:dbl, element #3=w6563:dbl, element #4=w6562:dbl, element #5=w6561:dbl, element #6=w6560:dbl, element #7=w6559:dbl, element #8=w6558:dbl, element #9=w6557:dbl, element #10=w6556:dbl, element #11=w6555:dbl, element #12=w6554:dbl, element #13=w6553:dbl, element #14=w6552:dbl, element #15=w6551:dbl, element #16=w6550:dbl, element #17=w6549:dbl)  [unwired: 17 in]
                    n4549 = global write "读配置文件全局.vi" "电池信息"(w6433) -> ()
                    n4550 = Index Array(array=w6435) -> (element #1=w6532:dbl, element #2=w6533:dbl, element #3=w6534:dbl, element #4=w6535:dbl, element #5=w6536:dbl, element #6=w6537:dbl, element #7=w6538:dbl, element #8=w6539:dbl, element #9=w6540:dbl, element #10=w6541:dbl, element #11=w6542:dbl, element #12=w6543:dbl, element #13=w6544:dbl, element #14=w6545:dbl, element #15=w6546:dbl, element #16=w6547:dbl, element #17=w6548:dbl)  [unwired: 17 in]
                    n4551 = Index Array(array=w6432) -> (element #1=w6527:dbl, element #2=w6526:dbl, element #3=w6525:dbl, element #4=w6524:dbl, element #5=w6523:dbl, element #6=w6522:dbl, element #7=w6521:dbl, element #8=w6520:dbl, element #9=w6519:dbl, element #10=w6518:dbl, element #11=w6517:dbl, element #12=w6516:dbl, element #13=w6515:dbl, element #14=w6514:dbl, element #15=w6513:dbl, element #16=w6512:dbl, element #17=w6511:dbl)  [unwired: 17 in]
                    n4552 = control-ref of="一级故障 3"() -> (w6510:refnum<vi>)
                    n4553 = control-ref of="一级故障 2"() -> (w6529:refnum<vi>)
                    n4554 = property class="Clust (严格)"(reference=w6529) -> (reference out=w6531:refnum<vi>, "Value"=w6530:T10)  [unwired: 1 in, 1 out]
                    n4555 = property class="Clust (严格)"(reference=w6510) -> (reference out=w6509:refnum<vi>, "Value"=w6528:T10)  [unwired: 1 in, 1 out]
                    n4556 = property class="Clust (严格)"(reference=w6495, "Value"=w6433) -> ()  [unwired: 1 in, 2 out]
                    n4557 = Bundle(cluster=w6530, "总电压过高"=w6532, "整组电压不均衡"=w6536, "SOC过高"=w6544, "单体电压过高"=w6540, "总电压过低"=w6533, "温度过高"=w6534, "温度过低"=w6535, "单组电压不均衡"=w6537, "整组温度不均衡"=w6538, "单组温度不均衡"=w6539, "单体电压过低"=w6541, "充电电流过高"=w6542, "放电电流过高"=w6543, "SOC过低"=w6545, "内阻过大"=w6546, "极柱温度过高"=w6547, "SOH过低"=w6548) -> (w6441:T10)
                    n4558 = Bundle(cluster=w6528, "总电压过高"=w6527, "整组电压不均衡"=w6523, "SOC过高"=w6515, "单体电压过高"=w6519, "总电压过低"=w6526, "温度过高"=w6525, "温度过低"=w6524, "单组电压不均衡"=w6522, "整组温度不均衡"=w6521, "单组温度不均衡"=w6520, "单体电压过低"=w6518, "充电电流过高"=w6517, "放电电流过高"=w6516, "SOC过低"=w6514, "内阻过大"=w6513, "极柱温度过高"=w6512, "SOH过低"=w6511) -> (w6440:T10)
                    n4559 = control-ref of="一级故障"() -> (w6568:refnum<vi>)
                    n4560 = property class="Clust (严格)"(reference=w6568) -> (reference out=w6566:refnum<vi>, "Value"=w6567:T10)  [unwired: 1 in, 1 out]
                    n4561 = Bundle(cluster=w6567, "总电压过高"=w6565, "整组电压不均衡"=w6561, "SOC过高"=w6553, "单体电压过高"=w6557, "总电压过低"=w6564, "温度过高"=w6563, "温度过低"=w6562, "单组电压不均衡"=w6560, "整组温度不均衡"=w6559, "单组温度不均衡"=w6558, "单体电压过低"=w6556, "充电电流过高"=w6555, "放电电流过高"=w6554, "SOC过低"=w6552, "内阻过大"=w6551, "极柱温度过高"=w6550, "SOH过低"=w6549) -> (w6442:T10)
                    n4562 = property class="Clust (严格)"(reference=w6566, "Value"=w6442) -> ()  [unwired: 1 in, 2 out]
                    n4563 = property class="Clust (严格)"(reference=w6531, "Value"=w6441) -> ()  [unwired: 1 in, 2 out]
                    n4564 = property class="Clust (严格)"(reference=w6509, "Value"=w6440) -> ()  [unwired: 1 in, 2 out]
                  }
                  frame #2 {
                    w6704 = 1 ("索引")
                    # "均衡计算-电压高阀值1级"
                    n4565 = call <vilib>:"Get Section Names.vi"("refnum"=w6719) -> ("section names"=w6720:string[], "refnum out"=w6724:T25)  [unwired: 8 in, 1 out]
                    n4566 = local read "从板号"() -> (w6702:u8)
                    n4567 = Delete From Array(array=w6720, length=2 ("长度"), index=0 ("索引")) -> (array with subset deleted=w6723:string[])  [unwired: 1 out]
                    n4568 = for {
                      tunnel: w6723 -> [w6740] mode=indexing
                      tunnel: w6724 -> [w6741]
                      tunnel: [w6733] -> w6701 mode=indexing
                      tunnel: [w6732] -> w6645
                      n4569 = call <vilib>:"Get Key Names.vi"("section"=w6740, "refnum"=w6741) -> ("key names"=w6732:string[], "refnum out"=w6739:T25)  [unwired: 6 in, 2 out]
                      n4570 = for {
                        tunnel: w6732 -> [w6745] mode=indexing
                        tunnel: w6740 -> [w6744]
                        tunnel: w6739 -> [w6743]
                        tunnel: [w6742] -> w6733 mode=indexing
                        n4571 = call-poly <vilib>:"Read Key.vi"("section"=w6744, "key"=w6745, "refnum"=w6743) -> ("value"=w6742:string)  [unwired: 5 in, 3 out]
                      }
                      n4572 = Index Array(array=w6733, index=0 ("索引")) -> (element=w6736:string)
                      n4573 = local read "输出数组"() -> (w6737:string[][])
                      n4574 = Decimal String To Number(string=w6736) -> (number=w6735:i32)  [unwired: 2 in, 1 out]
                      n4575 = Decrement(x=w6735) -> (x-1=w6731:i32)
                      n4576 = Replace Array Subset(array=w6737, new element=w6733, index (col)=w6731) -> (w6734:string[][])  [unwired: 1 in]
                      n4577 = local write "输出数组"(w6734) -> ()
                    }
                    "key names" <- w6645
                    n4578 = Decrement(x=w6702) -> (x-1=w6718:u8)
                    n4579 = Index Array(array=w6701, index (row)=w6718) -> (element=w6644:string[])  [unwired: 1 in]
                    n4580 = Search 1D Array(1D array=w6645, element="风机开启温度" ("元素")) -> (index of element=w6707:i32)  [unwired: 1 in]
                    n4581 = Search 1D Array(1D array=w6645, element="电压过高一级" ("元素"), start index (0)=w6707) -> (index of element=w6670:i32)
                    n4582 = Search 1D Array(1D array=w6645, element="均衡计算-电压高阀值1级" ("元素"), start index (0)=w6670) -> (index of element=w6668:i32)
                    n4583 = Array Subset(array=w6644, index=w6668, length=17 ("长度")) -> (w6667:string[])
                    n4584 = Decrement(x=w6707) -> (x-1=w6705:i32)
                    n4585 = Array Subset(array=w6644, index=w6704, length=w6705) -> (w6642:string[])
                    n4586 = Array Subset(array=w6644, index=w6670, length=21 ("长度")) -> (w6716:string[])
                    n4587 = Array Subset(array=w6645, index=w6704, length=w6705) -> (w6681:string[])
                    n4588 = Index Array(array=w6644, index=0 ("索引")) -> (element=w6676:string)
                    n4589 = Array Subset(array=w6644, index=w6707, length=7 ("长度")) -> (w6710:string[])
                    n4590 = for {
                      tunnel: w6667 -> [w6726] mode=indexing
                      tunnel: [w6725] -> w6666 mode=indexing
                      n4591 = Fract/Exp String To Number(string=w6726) -> (number=w6725:dbl)  [unwired: 3 in, 1 out]
                    }
                    n4592 = for {
                      tunnel: w6716 -> [w6728] mode=indexing
                      tunnel: [w6727] -> w6717 mode=indexing
                      n4593 = Fract/Exp String To Number(string=w6728) -> (number=w6727:dbl)  [unwired: 3 in, 1 out]
                    }
                    n4594 = Decimal String To Number(string=w6676) -> (number=w6675:i32)  [unwired: 2 in, 1 out]
                    n4595 = for {
                      tunnel: w6710 -> [w6730] mode=indexing
                      tunnel: [w6729] -> w6678 mode=indexing
                      n4596 = Fract/Exp String To Number(string=w6730) -> (number=w6729:dbl)  [unwired: 3 in, 1 out]
                    }
                    n4597 = global write "读配置文件全局2.vi" "从板板号"(w6675) -> ()
                    n4598 = Delete From Array(array=w6717, length=7 ("长度"), index=0 ("索引")) -> (deleted portion=w6680:dbl[], array with subset deleted=w6713:dbl[])
                    n4599 = Array To Cluster(array=w6678) -> (cluster=w6700:T26)
                    n4600 = global write "读配置文件全局2.vi" "加热控制参数"(w6678) -> ()
                    n4601 = Delete From Array(array=w6713, length=7 ("长度"), index=0 ("索引")) -> (deleted portion=w6673:dbl[], array with subset deleted=w6674:dbl[])
                    n4602 = local write "加热控制参数"(w6700) -> ()
                    n4603 = Array To Cluster(array=w6680) -> (cluster=w6684:T26)
                    n4604 = Array To Cluster(array=w6674) -> (cluster=w6682:T26)
                    n4605 = Array To Cluster(array=w6673) -> (cluster=w6683:T26)
                    n4606 = global write "读配置文件全局2.vi" "三级故障阀值"(w6674) -> ()
                    n4607 = global write "读配置文件全局2.vi" "一级故障阀值"(w6680) -> ()
                    n4608 = global write "读配置文件全局2.vi" "二级故障阀值"(w6673) -> ()
                    n4609 = local write "一级故障 6"(w6684) -> ()
                    n4610 = local write "一级故障 8"(w6682) -> ()
                    n4611 = local write "一级故障 7"(w6683) -> ()
                    n4612 = Search 1D Array(1D array=w6681, element="第1通道电压个数" ("元素")) -> (index of element=w6692:i32)  [unwired: 1 in]
                    n4613 = Search 1D Array(1D array=w6681, element="电压个数" ("元素")) -> ()  [unwired: 1 in, 1 out]
                    n4614 = Search 1D Array(1D array=w6681, element="温度个数" ("元素")) -> (index of element=w6694:i32)  [unwired: 1 in]
                    n4615 = Search 1D Array(1D array=w6681, element="第一个保险通道" ("元素")) -> (index of element=w6693:i32)  [unwired: 1 in]
                    n4616 = Array Subset(array=w6642, length=2 ("长度")) -> (w6689:string[])  [unwired: 1 in]
                    n4617 = Array Subset(array=w6642, index=w6694, length=2 ("长度")) -> (w6687:string[])
                    n4618 = Array Subset(array=w6642, index=w6693, length=20 ("长度")) -> (w6686:string[])
                    n4619 = Array Subset(array=w6642, index=w6692, length=20 ("长度")) -> (w6688:string[])
                    n4620 = Array Subset(array=w6642, length=27 ("长度")) -> (w6641:string[])  [unwired: 1 in]
                    n4621 = Insert Into Array(array=w6689, new element #1=w6688, new element #2=w6687, new element #3=w6686) -> ()  [unwired: 1 in, 1 out]
                    n4622 = Build Array(string[] ["电压个数", "温度个数", "第一个保险通道", "第一个保险位置", "第二个保险通道", "第二个保险位置", "第三个保险通道", "第三个保险位置", "第四个保险通道", "第四个保险位置", "第五个保险通道", "第五个保险位置", "第六个保险通道", "第六个保险位置", "第七个保险通道", "第七个保险位置", "第八个保险通道", "第八个保险位置", "第九个保险通道", "第九个保险位置", "第十个保险通道", "第十个保险位置", "第1通道电压个数", "第2通道电压个数", "第3通道电压个数", "第4通道电压个数", "第5通道电压个数"], w6641) -> (w6685:string[][])
                    n4623 = global write "读配置文件全局2.vi" "表格"(w6641) -> ()
                    n4624 = Index Array(array=w6666) -> (element #1=w6663:dbl, element #2=w6662:dbl, element #3=w6661:dbl, element #4=w6660:dbl, element #5=w6659:dbl, element #6=w6658:dbl, element #7=w6657:dbl, element #8=w6656:dbl, element #9=w6655:dbl, element #10=w6654:dbl, element #11=w6653:dbl, element #12=w6652:dbl, element #13=w6651:dbl, element #14=w6650:dbl, element #15=w6649:dbl, element #16=w6648:dbl, element #17=w6647:dbl, element #18=w6646:dbl)  [unwired: 18 in]
                    n4625 = Transpose 2D Array(2D array=w6685) -> (transposed array=w6679:string[][])
                    n4626 = local write "项目信息 2"(w6679) -> ()
                    n4627 = local read "均衡参数"() -> (w6665:T17)
                    n4628 = Bundle(cluster=w6665, "充电结束电压(90%)"=w6656, "充电结束电压(91%)"=w6655, "充电结束电压(92%)"=w6654, "充电结束电压(93%)"=w6653, "充电结束电压(94%)"=w6652, "均衡计算-电压高阀值1级"=w6663, "均衡计算-电压高阀值2级"=w6662, "均衡计算-电压低阀值1级"=w6661, "均衡计算-电压低阀值2级"=w6660, "均衡计算-最低电压阀值"=w6659, "均衡停止-最低电压阀值"=w6658, "均衡计算-电压极差阀值"=w6657, "充电结束电压(95%)"=w6651, "充电结束电压(96%)"=w6650, "充电结束电压(97%)"=w6649, "充电结束电压(98%)"=w6648, "充电结束电压(99%)"=w6647, "充电结束电压(100%)"=w6646) -> (w6664:T17)
                    n4629 = local write "均衡参数"(w6664) -> ()
                  }
                  frame #3 {
                    n4630 = call <vilib>:"Unset Busy.vi"() -> ()  [unwired: 11 in, 1 out]
                    n4631 = Build Array("读取完成") -> (w6749:string[])
                    n4632 = property on="全部写入" class="Bool (严格)"("DisabledEnum"=0) -> ()  [unwired: 2 in, 2 out]
                    n4633 = call "表格编辑.vi"("新元素/子数组"=w6749, "活动单元格:单元格背景色"=u32 6618880, "MCListbox引用句柄"=w6746) -> ()  [unwired: 9 out]
                  }
                }
              }
            }
          }
        }
      }
      frame Error {
      }
    }
  }
  n4634 = Release Queue(queue=w28, force destroy? (F)=TRUE ("强制销毁？(F)"), error in (no error)=w27) -> (error out=w30:errorcluster)  [unwired: 2 out]
  n4635 = call <vilib>:"Clear Errors.vi"("error in (no error)"=w30) -> ()  [unwired: 7 out]
  n4636 = local write "面板选择"(T7."读写参数" ("面板选择")) -> ()
  n4637 = Release Queue(queue=w34, force destroy? (F)=TRUE ("强制销毁？(F)"), error in (no error)=w33) -> (error out=w31:errorcluster)  [unwired: 2 out]
  n4638 = call <vilib>:"Clear Errors.vi"("error in (no error)"=w31) -> ()  [unwired: 7 out]
